vi "Distance-Velocity Calculation RT.vi"(0 "First FFT":dbl[](array[numeric]), 5 "Second FFT":dbl[](array[numeric]), 6 "Windowing":T1(ring), 8 "first FFT bin":i32=10, 9 "Sample Rate (S/s)":dbl=50000000.0, 10 "last FFT bin":i32=255) -> (11 "F_rise":dbl, 12 "maxbin_firstFFT":i32, 13 "maxbin_secondFFT":i32, 14 "Distance (m)":dbl, 16 "f_mean":dbl, 17 "F_fall":dbl, 19 "Velocity (m/s)":dbl)   [LabVIEW 2014]
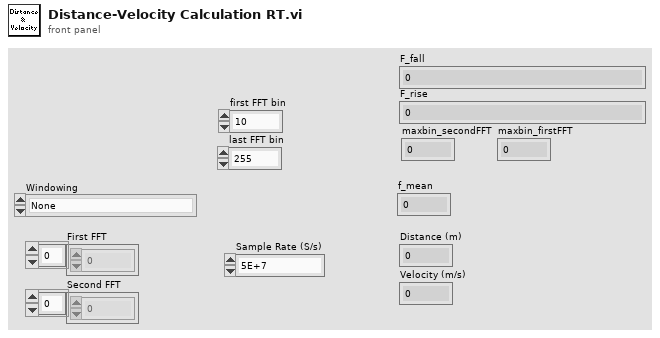
[diagram p1: front panel]
types:
  T1 = enum16{"None", "Hanning", "Hamming", "Blackman", "Blackman-Harris"}
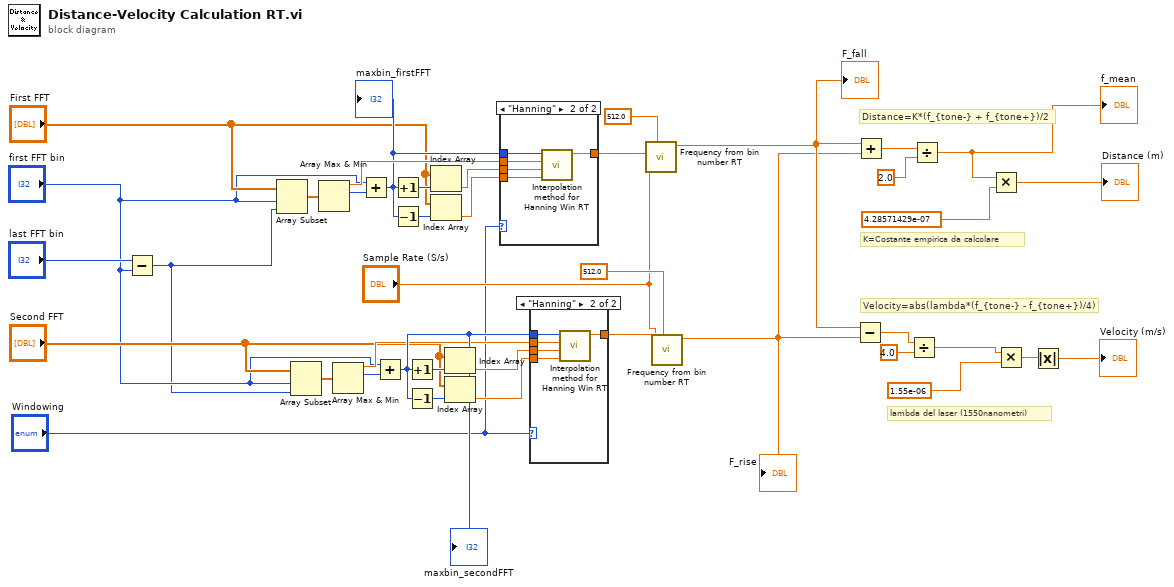
[diagram p0: block diagram]
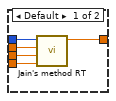
[diagram p2: hidden frame]
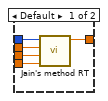
[diagram p3: hidden frame]
diagram:
  # "Velocity=abs(lambda*(f_{tone-} - f_{tone+})/4)"
  # "Distance=K*(f_{tone-} + f_{tone+})/2"
  # "lambda del laser (1550nanometri)"
  # "K=Costante empirica da calcolare"
  n1 = Subtract(x="last FFT bin", y="first FFT bin") -> (x-y=w2:i32)
  n2 = Array Subset(array="First FFT", index="first FFT bin", length=w2) -> (w40:dbl[])
  n3 = Array Subset(array="Second FFT", index="first FFT bin", length=w2) -> (w39:dbl[])
  n4 = Array Max & Min(array=w40) -> (max value=w36:dbl, max index (indices)=w38:i32)  [unwired: 2 out]
  n5 = Array Max & Min(array=w39) -> (max value=w24:dbl, max index (indices)=w37:i32)  [unwired: 2 out]
  n6 = Add(x="first FFT bin", y=w38) -> (x+y=w33:i32)
  "maxbin_firstFFT" <- w33
  n7 = Add(x="first FFT bin", y=w37) -> (x+y=w25:i32)
  "maxbin_secondFFT" <- w25
  n8 = Increment(x=w33) -> (x+1=w35:i32)
  n9 = Decrement(x=w33) -> (x-1=w32:i32)
  n10 = Increment(x=w25) -> (x+1=w29:i32)
  n11 = Decrement(x=w25) -> (x-1=w27:i32)
  n12 = Index Array(array="First FFT", index=w35) -> (element=w34:dbl)
  n13 = Index Array(array="First FFT", index=w32) -> (element=w30:dbl)
  n14 = Index Array(array="Second FFT", index=w29) -> (element=w28:dbl)
  n15 = Index Array(array="Second FFT", index=w27) -> (element=w26:dbl)
  n16 = case shown="\"Hanning\"" "Windowing" {
    tunnel: w36 -> [w45 w47]
    tunnel: w34 -> [w44 w48]
    tunnel: w33 -> [w43 w46]
    tunnel: w30 -> [w42 w49]
    tunnel: [w41 w50] -> w22
    frame Default {
      n17 = call "Jain's method RT.vi"("Prev Amp"=w42, "Next Amp"=w44, "Max Amp"=w45, "Max Bin"=w43) -> ("Bin"=w41:dbl)  [unwired: 7 in]
    }
    frame "Hanning" {
      n18 = call "Interpolation method for Hanning Win RT.vi"("Prev Amp"=w49, "Next Amp"=w48, "Max Amp"=w47, "Max Bin"=w46) -> ("Bin"=w50:dbl)  [unwired: 7 in]
    }
  }
  n19 = case shown="\"Hanning\"" "Windowing" {
    tunnel: w28 -> [w55 w58]
    tunnel: w26 -> [w54 w59]
    tunnel: w25 -> [w53 w56]
    tunnel: w24 -> [w52 w57]
    tunnel: [w51 w60] -> w21
    frame Default {
      n20 = call "Jain's method RT.vi"("Prev Amp"=w54, "Next Amp"=w55, "Max Amp"=w52, "Max Bin"=w53) -> ("Bin"=w51:dbl)  [unwired: 7 in]
    }
    frame "Hanning" {
      n21 = call "Interpolation method for Hanning Win RT.vi"("Prev Amp"=w59, "Next Amp"=w58, "Max Amp"=w57, "Max Bin"=w56) -> ("Bin"=w60:dbl)  [unwired: 7 in]
    }
  }
  n22 = call "Frequency from bin number RT.vi"("FFT size"=512.0, "Bin number"=w22, "Sample Rate (S/s)"="Sample Rate (S/s)") -> ("Detected Frequency (Hz)"=w9:dbl)  [unwired: 8 in]
  "F_fall" <- w9
  n23 = call "Frequency from bin number RT.vi"("FFT size"=512.0, "Bin number"=w21, "Sample Rate (S/s)"="Sample Rate (S/s)") -> ("Detected Frequency (Hz)"=w8:dbl)  [unwired: 8 in]
  "F_rise" <- w8
  n24 = Subtract(x=w9, y=w8) -> (x-y=w13:dbl)
  n25 = Add(x=w9, y=w8) -> (x+y=w18:dbl)
  n26 = Divide(x=w13, y=4.0) -> (x/y=w11:dbl)
  n27 = Divide(x=w18, y=2.0) -> (x/y=w16:dbl)
  "f_mean" <- w16
  n28 = Multiply(x=w16, y=4.28571429e-07) -> (x*y=→"Distance (m)":dbl)
  n29 = Multiply(x=w11, y=1.55e-06) -> (x*y=w7:dbl)
  n30 = Absolute Value(x=w7) -> (abs(x)=→"Velocity (m/s)":dbl)
